vi "initCOMPORT.vi"(8 "error IO":errorcluster, 11 "OUT COM 2":refnum<visa-resource-name>) -> (0 "error out":errorcluster, 3 "OUT COM 3":refnum<visa-resource-name>)   [LabVIEW 2017]
uses:
  mWorkToolkit/libSerial/stateSerialUltra.ctl
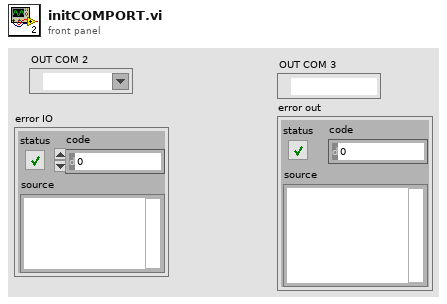
[diagram p1: front panel]
types:
  T1 = enum16{"FindCom", "DelayCheckError", "InitCom", "WriteTest", "SetBuffer"}
  T2 = typedef "stateSerialUltra.ctl" = enum16{"findCOM", "Init", "CheckConnect", "Read", "Write", "exit"}
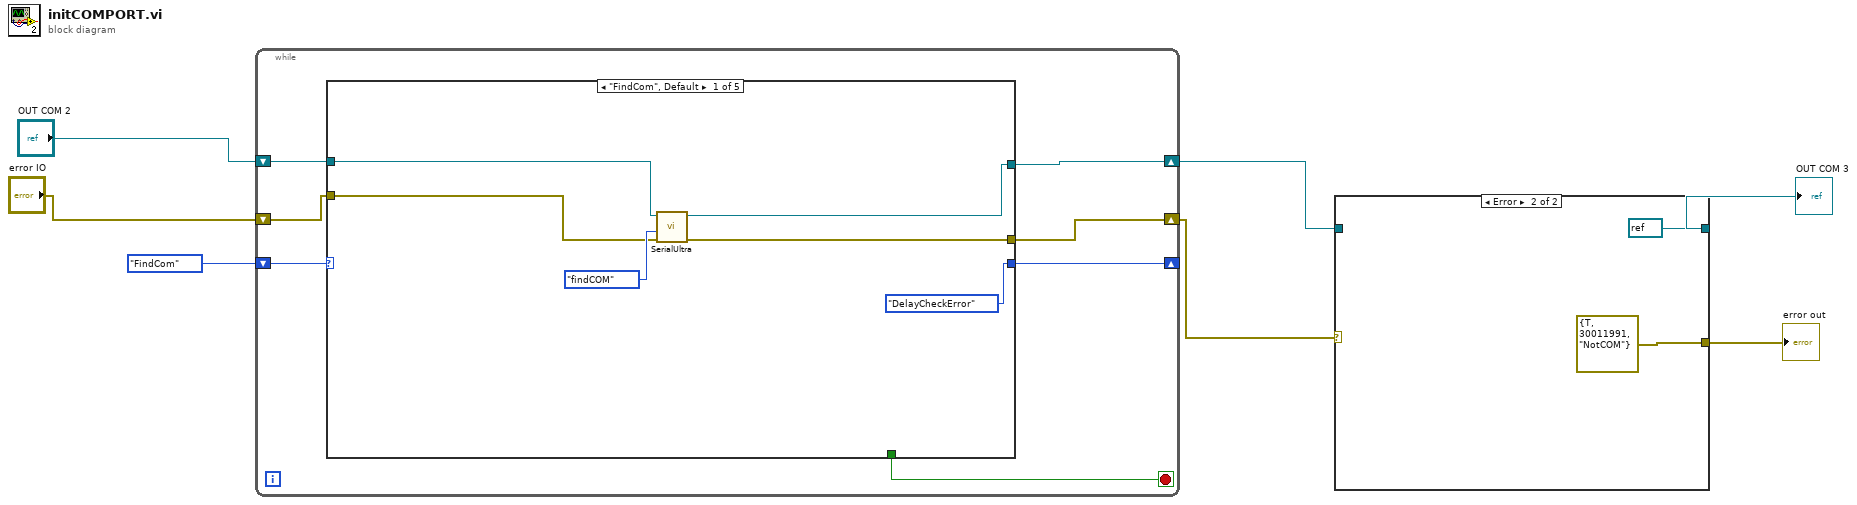
[diagram p0: block diagram]
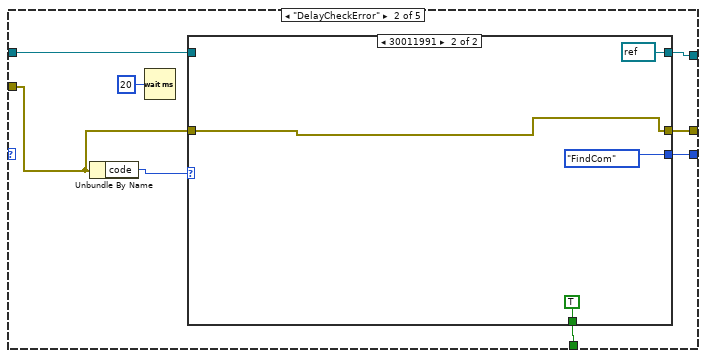
[diagram p3: hidden frame]
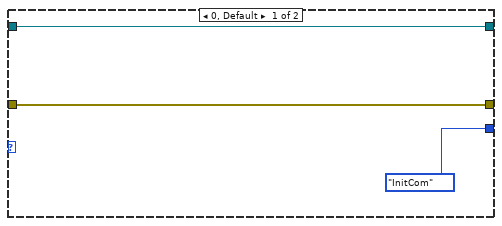
[diagram p4: hidden frame]
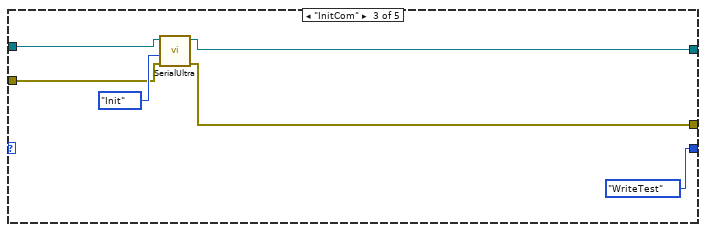
[diagram p5: hidden frame]
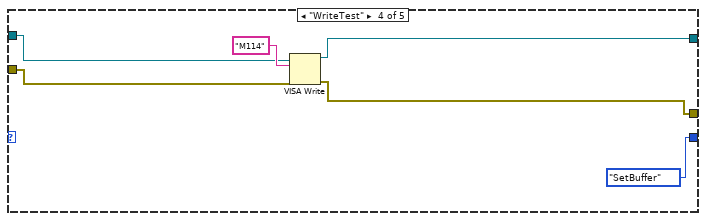
[diagram p6: hidden frame]
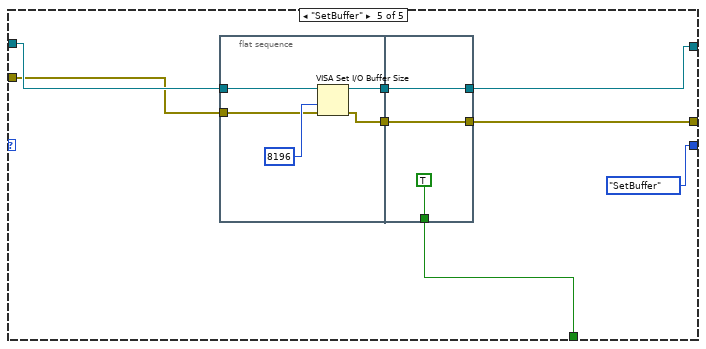
[diagram p7: hidden frame]
diagram:
  n1 = while {
    shift-right: [w10] -> _
    shift-left: T1."FindCom" ("State") -> [w14]
    shift-right: [w11] -> w2
    shift-left: "OUT COM 2" -> [w13]
    shift-right: [w12] -> w5
    shift-left: "error IO" -> [w8]
    stop <- w9 stop-if-true
    n2 = case shown="\"FindCom\", Default" w14 {
      tunnel: w13 -> [w19 w24 w40 w46 w53]
      tunnel: [w18 w27 w37 w43 w55] -> w12
      tunnel: w8 -> [w17 w21 w39 w45 w52]
      tunnel: [w16 w25 w38 w44 w54] -> w11
      tunnel: [T1."DelayCheckError" ("State") w26 T1."WriteTest" ("State") T1."SetBuffer" ("State") T1."SetBuffer" ("State")] -> w10
      tunnel: [_ w23 _ _ w48] -> w9
      frame "FindCom", Default {
        n3 = call "SerialUltra.vi"("error in"=w17, "State"=stateSerialUltra."findCOM", "IN COM"=w19) -> ("error out"=w18:errorcluster, "OUT COM 2"=w16:refnum<visa-resource-name>)  [unwired: 4 in, 3 out]
      }
      frame "DelayCheckError" {
        n4 = Unbundle By Name(w21) -> ("code"=w22:i32)
        n5 = Wait (ms)(milliseconds to wait=u32 20) -> ()  [unwired: 1 out]
        n6 = case shown="30011991" w22 {
          tunnel: [w29 w32] -> w27
          tunnel: [T1."InitCom" ("State") T1."FindCom" ("State")] -> w26
          tunnel: [_ TRUE ("OK")] -> w23
          tunnel: [w30 refnum<visa-resource-name> refnum ("OUT COM 2")] -> w25
          tunnel: w24 -> [w30 _]
          tunnel: w21 -> [w29 w32]
          frame 0, Default {
          }
          frame 30011991 {
          }
        }
      }
      frame "InitCom" {
        n7 = call "SerialUltra.vi"("error in"=w39, "State"=stateSerialUltra."Init", "IN COM"=w40) -> ("error out"=w37:errorcluster, "OUT COM 2"=w38:refnum<visa-resource-name>)  [unwired: 4 in, 3 out]
      }
      frame "WriteTest" {
        n8 = VISA Write(VISA resource name=w46, write buffer="M114", error in (no error)=w45) -> (VISA resource name out=w44:refnum<visa-resource-name>, error out=w43:errorcluster)  [unwired: 1 out]
      }
      frame "SetBuffer" {
        n9 = flat-sequence {
          tunnel: w53 -> [w57]
          tunnel: w52 -> [w56]
          tunnel: [w59] -> w50
          tunnel: [w58] -> w49
          tunnel: [w62] -> w54
          tunnel: [w63] -> w55
          tunnel: w50 -> [w63]
          tunnel: w49 -> [w62]
          tunnel: [TRUE] -> w48
          frame #0 {
            n10 = VISA Set I/O Buffer Size(VISA resource name=w57, size (4096)=u32 8196, error in (no error)=w56) -> (VISA resource name out=w58:refnum<visa-resource-name>, error out=w59:errorcluster)  [unwired: 1 in]
          }
          frame #1 {
          }
        }
      }
    }
  }
  n11 = case shown="Error" w5 {
    selector: w5 -> [w65 _]
    tunnel: [w65 errorcluster {"status"=TRUE, "code"=30011991, "source"="NotCOM"} ("error IO")] -> w4
    tunnel: [w64 refnum<visa-resource-name> refnum ("OUT COM 2")] -> w3
    tunnel: w2 -> [w64 _]
    frame No Error {
    }
    frame Error {
    }
  }
  "OUT COM 3" <- w3
  "error out" <- w4
